vi "FSM_new.vi"() -> ()   [LabVIEW 2016]
panel:
  out "note":string
  out "Waveform Graph 2":dbl[](graph)
  out "Select traing signal":i32
  out "Saved Target":fxp<+/-,32,8>[][](array[numeric])
  out "Number of Signals":i32
  out "Signal Captured":fxp<+/-,32,8>[][](array[numeric])
  in  "Signal Capture":bool
  out "Final Error":fxp<+/-,32,8>
  out "Waveform Graph":dbl[](graph)
  in  "Inference":bool
  in  "Training":bool
  out "Enum":T1(ring)
  out "Weights_oX":fxp<+/-,32,8>[][](array[numeric])
  out "Weights_hX":fxp<+/-,32,8>[][](array[numeric])
  out "Outputs_oX":fxp<+/-,32,8>[](array[numeric])
  out "Outputs_hX":fxp<+/-,32,8>[](array[numeric])
  in  "Target 6":fxp<+/-,32,8>
  in  "Target 5":fxp<+/-,32,8>
  in  "Target 7":fxp<+/-,32,8>
  in  "Target 8":fxp<+/-,32,8>
  in  "Learning rate":fxp<+/-,32,8>
  in  "Offset 2":fxp<+/-,32,8>
  in  "Offset 1":fxp<+/-,32,8>
  out "Random values generated":bool
  out "Training end":bool
  in  "Target 4":fxp<+/-,32,8>
  in  "Target 3":fxp<+/-,32,8>
  in  "Target 2":fxp<+/-,32,8>
  in  "Target 1":fxp<+/-,32,8>
  in  "Stop":bool
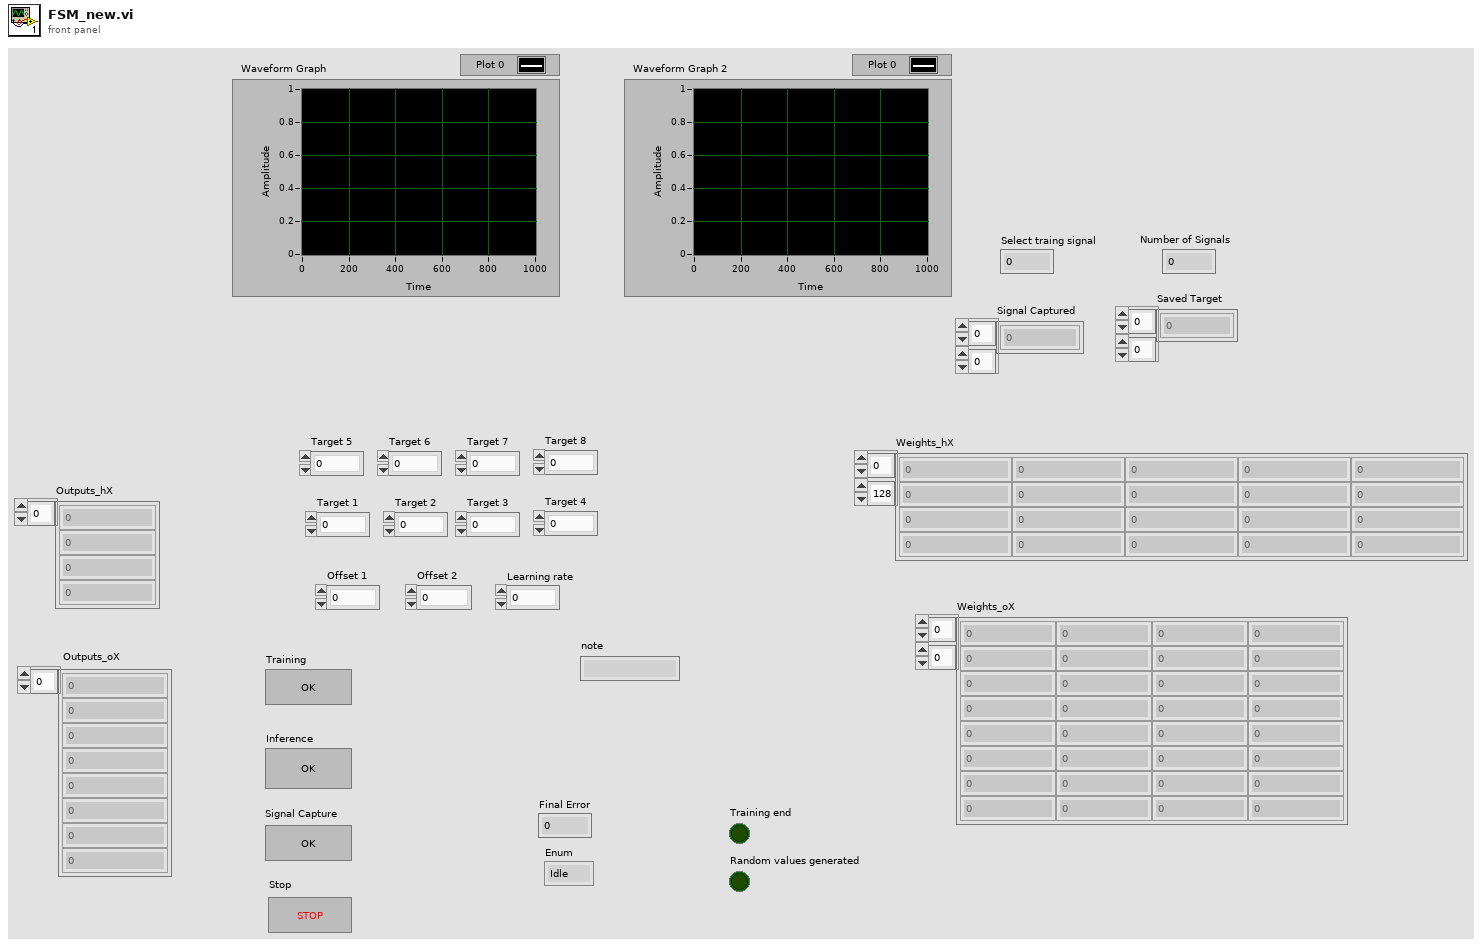
[diagram p1: front panel]
types:
  T1 = enum16{"Idle", "Generate weights", "Training mode", "Inference mode"}
  T2 = enum16{"Idle", "Generate weights", "Training mode", "Inference mode", "Signal Capture"}
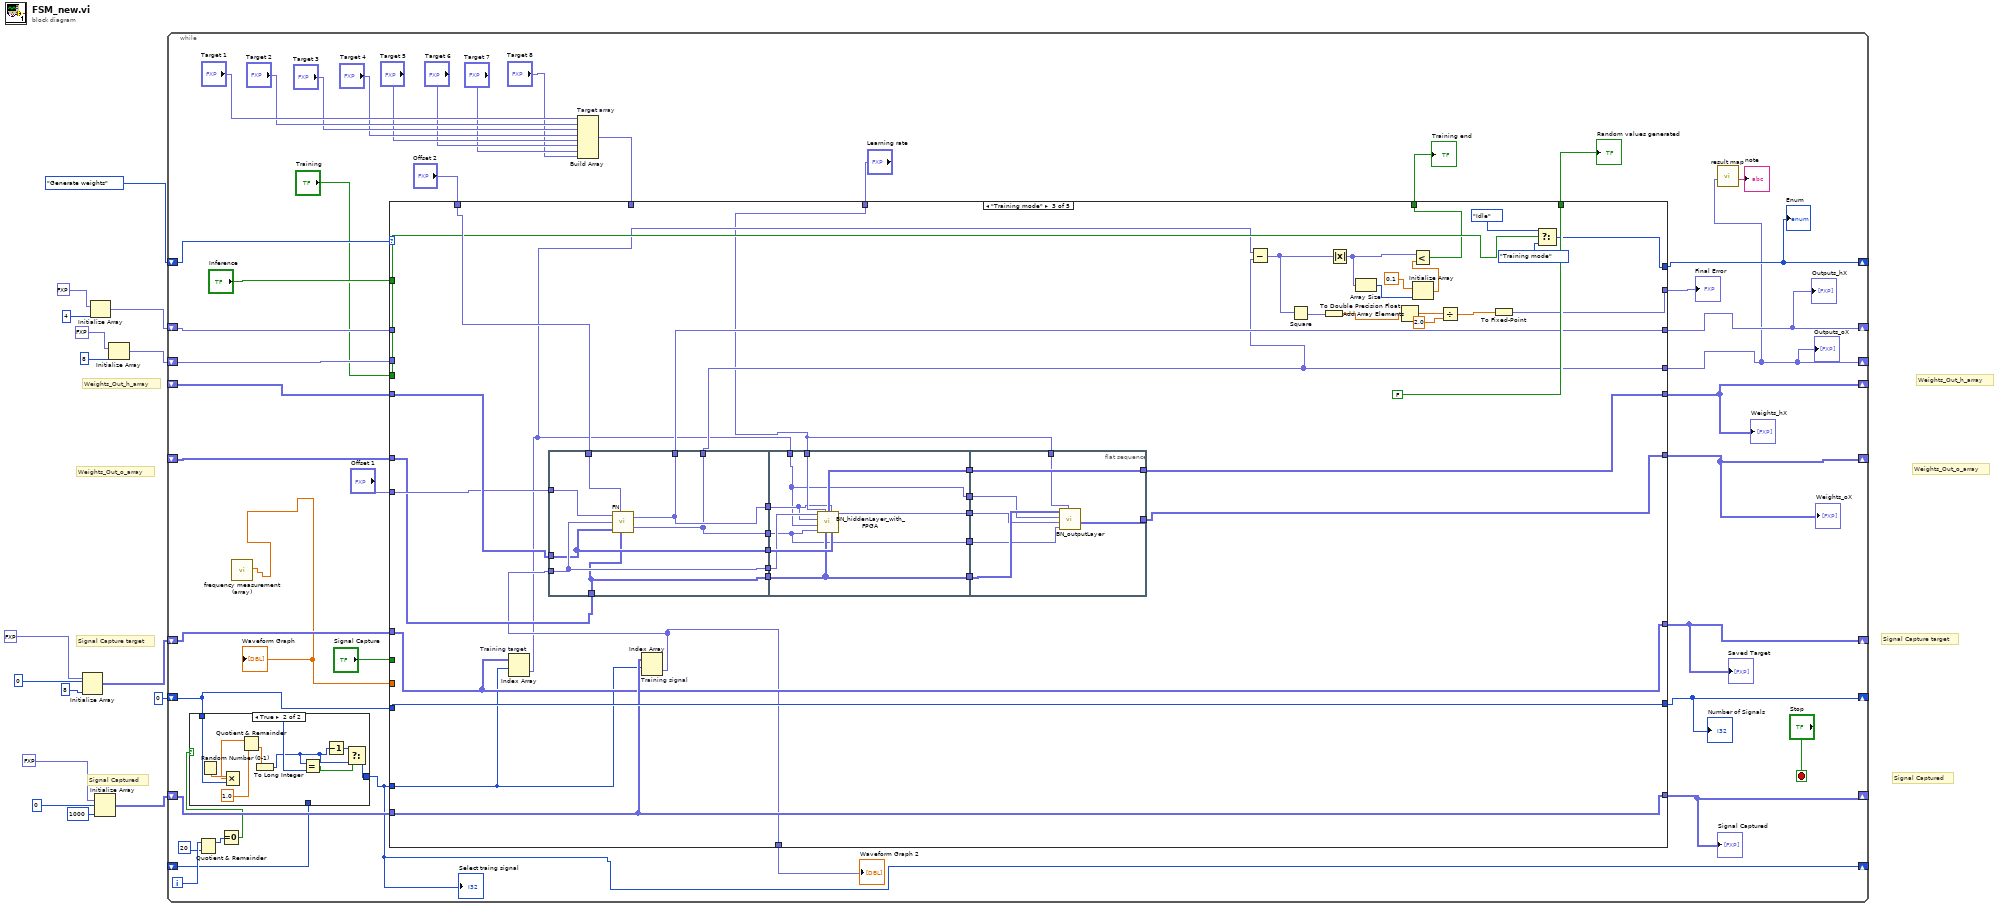
[diagram p0: block diagram]
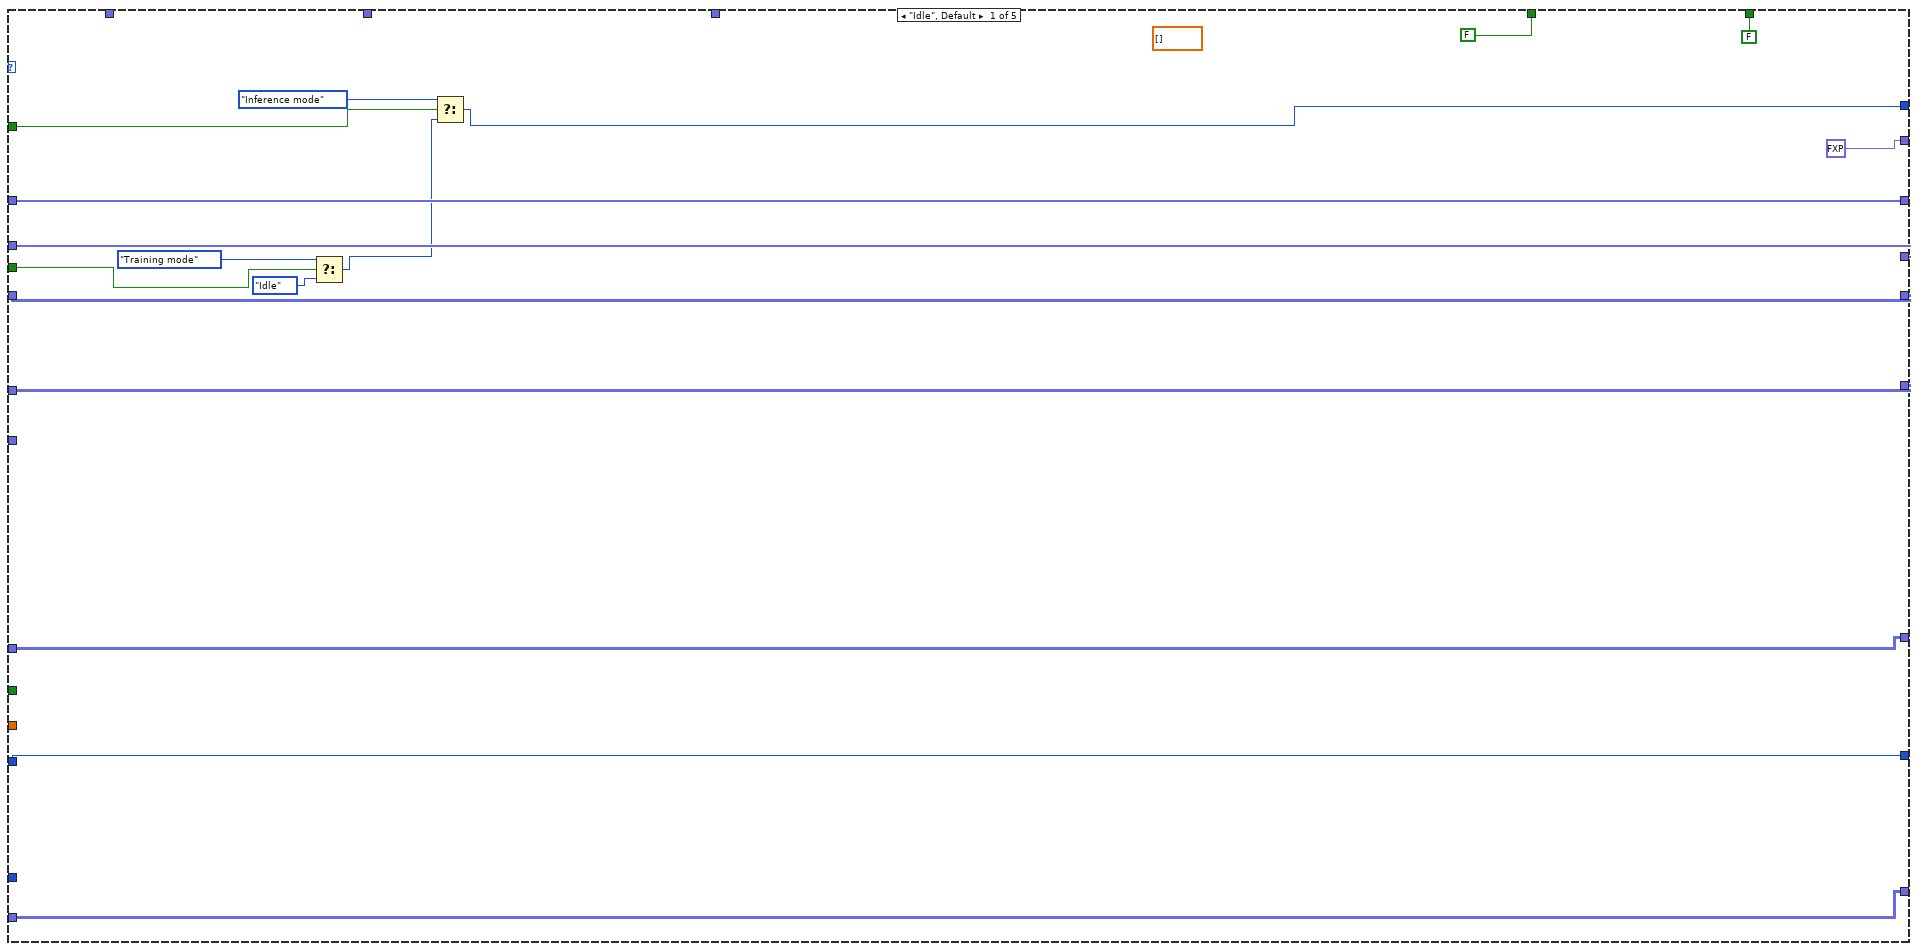
[diagram p3: hidden frame]
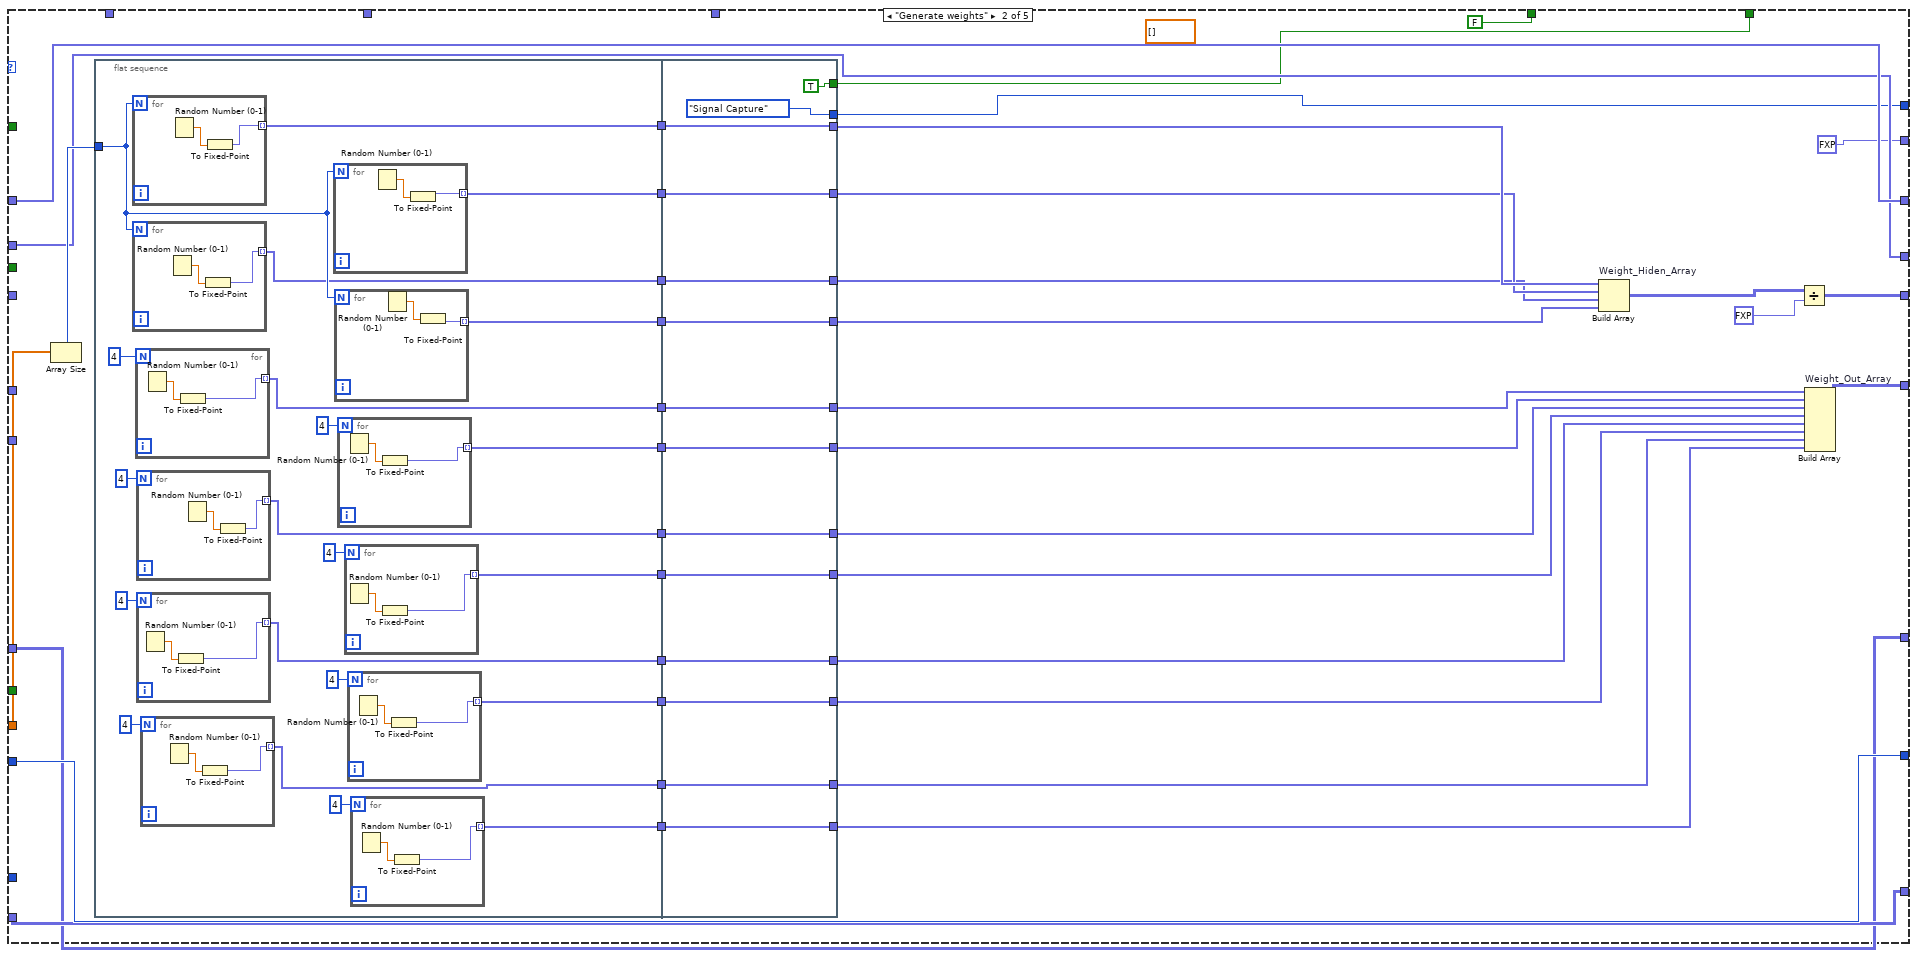
[diagram p4: hidden frame]
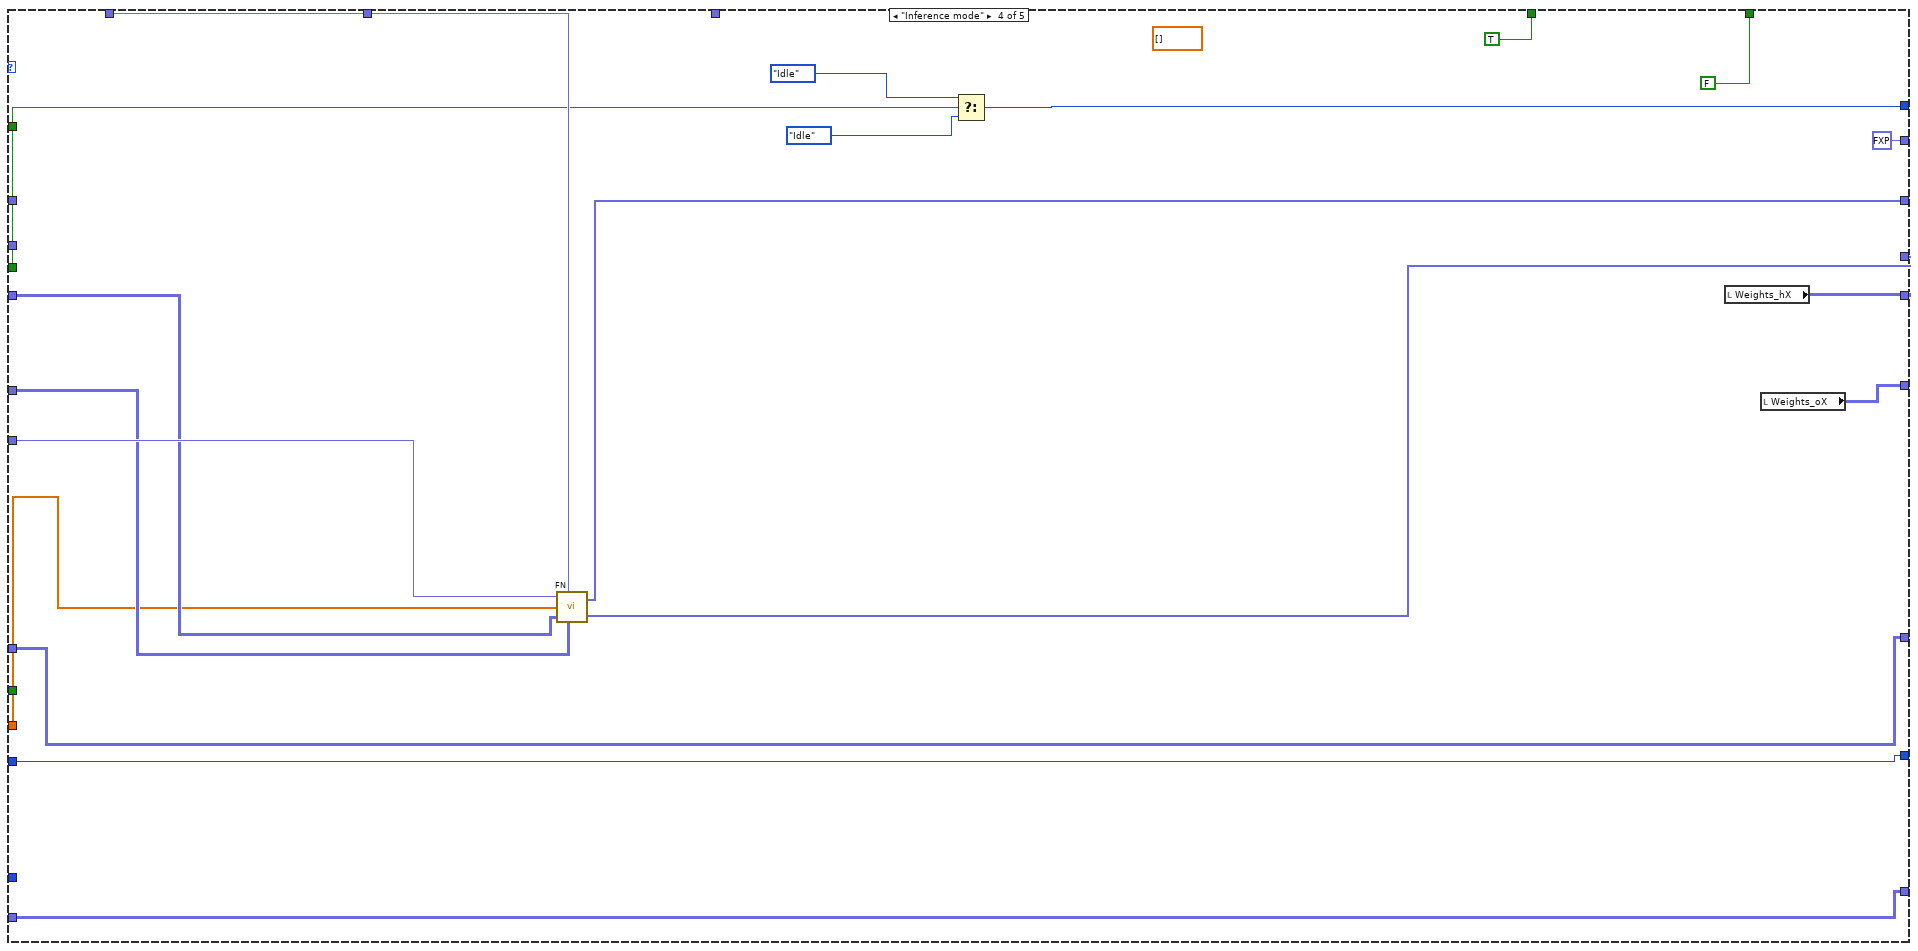
[diagram p5: hidden frame]
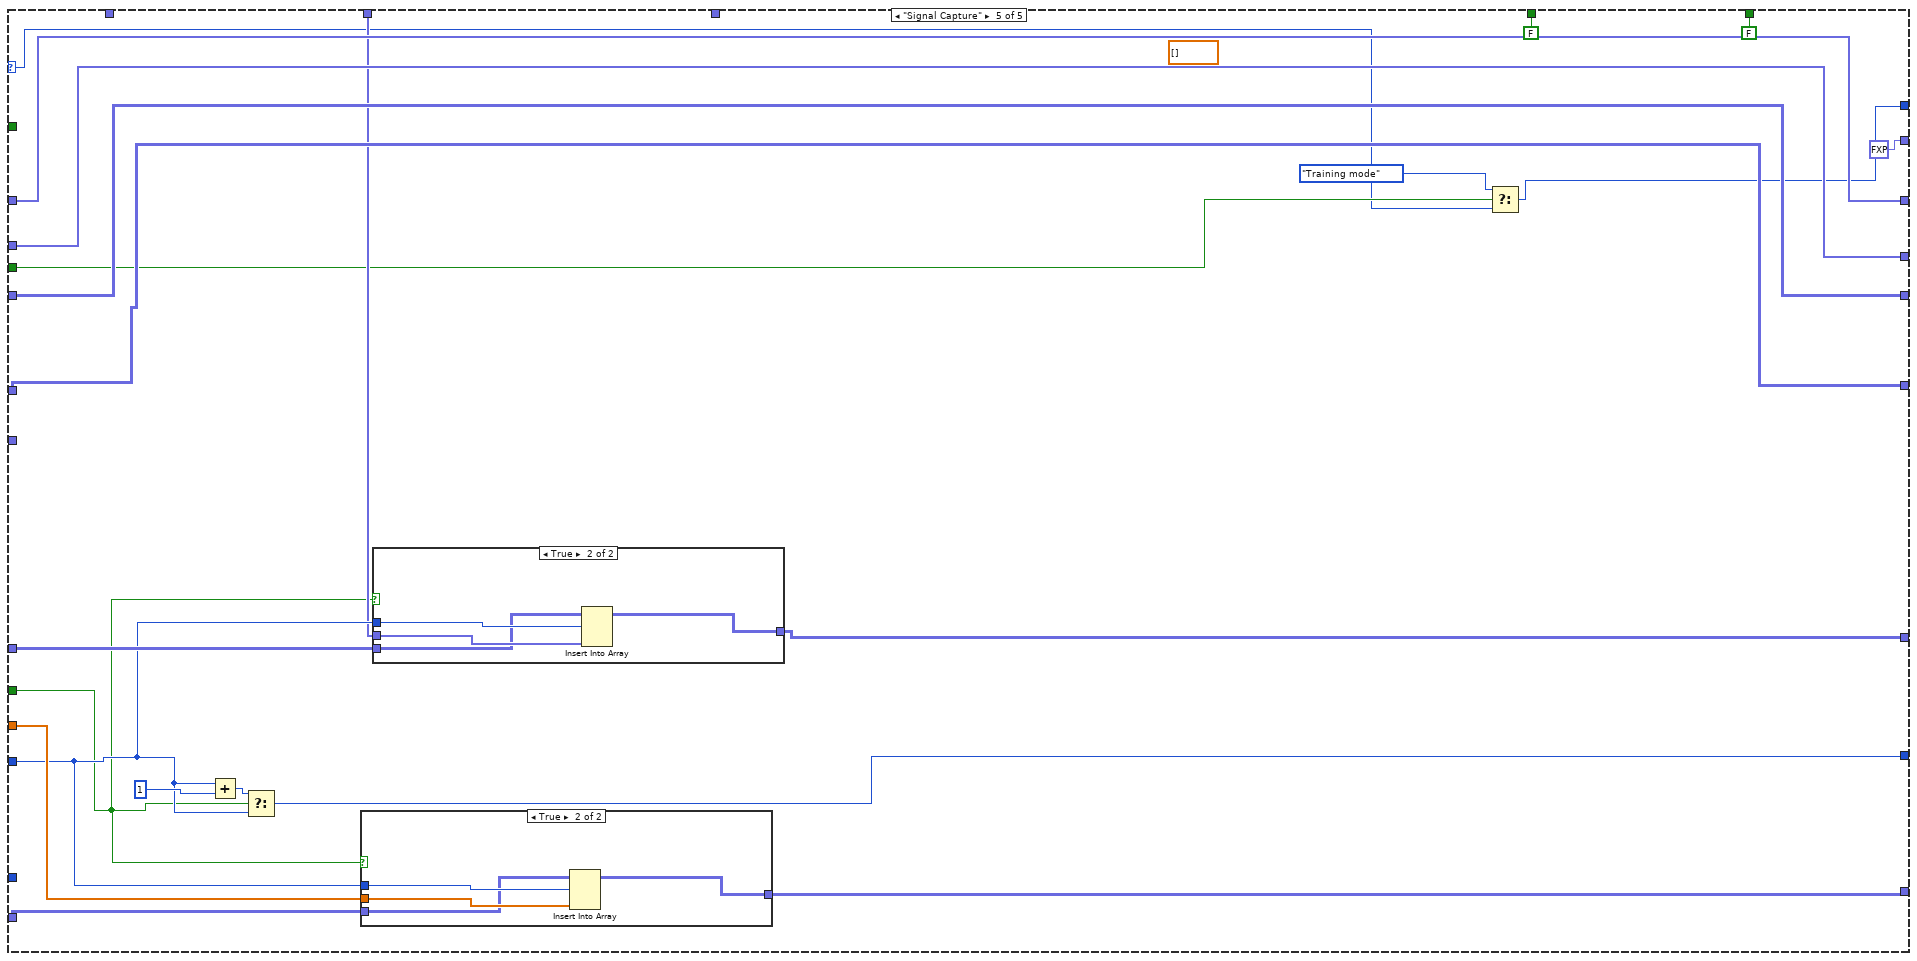
[diagram p6: hidden frame]
diagram:
  # "Signal Captured"
  # "Signal Capture target"
  # "Signal Captured"
  # "Signal Capture target"
  # "Weights_Out_o_array"
  # "Weights_Out_h_array"
  # "Weights_Out_o_array"
  # "Weights_Out_h_array"
  n1 = Initialize Array(fxp<+,32,8> 0.0, 0, 8 ("dimension size")) -> (w1:fxp<+,32,8>[][])
  n2 = Initialize Array(fxp<+,32,8> 0.0, 4) -> (w15:fxp<+,32,8>[])
  n3 = Initialize Array(fxp<+/-,32,8> 0.0, 0, 1000 ("dimension size")) -> (w6:fxp<+/-,32,8>[][])
  n4 = Initialize Array(fxp<+,32,8> 0.0, 8) -> (w10:fxp<+,32,8>[])
  n5 = while {
    shift-right: [w39] -> _
    shift-left: T2."Generate weights" -> [w56]
    shift-right: [w44] -> _
    shift-left: _ -> [w43]
    shift-right: [w45] -> _
    shift-left: _ -> [w42]
    shift-right: [w38] -> _
    shift-left: w15 -> [w41]
    shift-right: [w18] -> _
    shift-left: w10 -> [w40]
    shift-right: [w32] -> _
    shift-left: 0 -> [w25]
    shift-right: [w31] -> _
    shift-left: w6 -> [w30]
    shift-right: [w28] -> _
    shift-left: w1 -> [w29]
    shift-right: [w19] -> _
    shift-left: _ -> [w20]
    i -> [w24]
    stop <- "Stop" stop-if-true
    n6 = Quotient & Remainder(x=w24, y=20) -> (x-y*floor(x/y)=w22:i32)  [unwired: 1 out]
    n7 = Equal To 0?(x=w22) -> (x = 0?=w21:bool)
    n8 = case shown="True" w21 {
      tunnel: w25 -> [_ w66]
      tunnel: [w61 w62] -> w19
      tunnel: w20 -> [w61 _]
      frame False {
      }
      frame True {
        n9 = Random Number (0-1)() -> (number: 0 to 1=w70:dbl)
        n10 = Multiply(x=w70, y=w66) -> (x*y=w69:dbl)
        n11 = Quotient & Remainder(x=w69, y=1.0) -> (floor(x/y)=w67:dbl)  [unwired: 1 out]
        n12 = To Long Integer(number=w67) -> (32bit integer=w63:i32)
        n13 = Equal?(x=w63, y=w66) -> (x = y?=w65:bool)
        n14 = Decrement(x=w63) -> (x-1=w64:i32)
        n15 = Select(t=w64, s=w65, f=w63) -> (s? t:f=w62:i32)
      }
    }
    "Select traing signal" <- w19
    n16 = call "frequency measurement (array).vi"() -> ("real part of fft array"=w26:dbl[])  [unwired: 11 in]
    "Waveform Graph" <- w26
    n17 = Build Array "Target array"("Target 1", "Target 2", "Target 3", "Target 4", "Target 5", "Target 6", "Target 7", "Target 8") -> (w47:fxp<+/-,32,8>[])
    n18 = case shown="\"Training mode\"" w56 {
      selector: w56 -> [_ _ _ _ w271]
      tunnel: [w75 w89 w214 w257 w273] -> w39
      tunnel: [FALSE w97 FALSE FALSE FALSE] -> w46
      tunnel: "Offset 1" -> [_ _ w225 w267 _]
      tunnel: "Offset 2" -> [_ _ w224 w268 _]
      tunnel: "Learning rate" -> [_ _ w190 _ _]
      tunnel: w47 -> [_ _ _ _ w276]
      tunnel: [w83 w100 w223 w266 w290] -> w38
      tunnel: [w82 w99 w217 w265 w289] -> w18
      tunnel: w26 -> [_ w98 _ w254 w281]
      tunnel: [w85 w94 w198 w263 w288] -> w44
      tunnel: [w84 w101 w186 w262 w287] -> w45
      tunnel: w43 -> [w85 _ w226 w261 w288]
      tunnel: w42 -> [w84 _ w205 w260 w287]
      tunnel: w41 -> [w83 w100 _ _ w290]
      tunnel: w40 -> [w82 w99 _ _ w289]
      tunnel: "Training" -> [w80 _ w209 w256 w272]
      tunnel: [FALSE FALSE w208 TRUE FALSE] -> w37
      tunnel: "Inference" -> [w77 _ _ _ _]
      tunnel: [fxp<+,32,8> 0.0 fxp<+,32,8> 0.0 w197 fxp<+,32,8> 0.0 fxp<+,32,8> 0.0] -> w34
      tunnel: "Signal Capture" -> [_ _ _ _ w275]
      tunnel: [w73 w92 w204 w252 w282] -> w32
      tunnel: w25 -> [w73 w92 w204 w252 w277]
      tunnel: [w74 w91 w203 w251 w280] -> w31
      tunnel: w30 -> [w74 w91 w203 w251 w279]
      tunnel: w29 -> [w72 w90 w202 w250 w278]
      tunnel: [w72 w90 w202 w250 w274] -> w28
      tunnel: w19 -> [_ _ w199 _ _]
      tunnel: [_ _ w201 _ _] -> w27
      frame "Idle", Default {
        (unwired) dbl[] [] ("Error_out")
        n19 = Select(t=T1."Training mode", s=w80, f=T1."Idle") -> (s? t:f=w76:T1)
        n20 = Select(t=T1."Inference mode", s=w77, f=w76) -> (s? t:f=w75:T1)
      }
      frame "Generate weights" {
        (unwired) dbl[] [] ("Error_out")
        n21 = Array Size(array=w98) -> (size(s)=w126:i32)
        n22 = flat-sequence {
          tunnel: w126 -> [w147]
          tunnel: [w146] -> w125
          tunnel: [w145] -> w124
          tunnel: [w144] -> w123
          tunnel: [w143] -> w122
          tunnel: [w142] -> w121
          tunnel: [w141] -> w120
          tunnel: [w140] -> w119
          tunnel: [w139] -> w118
          tunnel: [w138] -> w117
          tunnel: [w137] -> w116
          tunnel: [w136] -> w115
          tunnel: [w135] -> w114
          tunnel: [TRUE] -> w97
          tunnel: w125 -> [w184]
          tunnel: [w184] -> w113
          tunnel: w124 -> [w183]
          tunnel: [w183] -> w111
          tunnel: w123 -> [w182]
          tunnel: [w182] -> w102
          tunnel: w122 -> [w181]
          tunnel: [w181] -> w104
          tunnel: w121 -> [w180]
          tunnel: [w180] -> w106
          tunnel: w120 -> [w179]
          tunnel: [w179] -> w108
          tunnel: w119 -> [w178]
          tunnel: [w178] -> w112
          tunnel: w118 -> [w177]
          tunnel: [w177] -> w110
          tunnel: w117 -> [w176]
          tunnel: [w176] -> w103
          tunnel: w116 -> [w175]
          tunnel: [w175] -> w105
          tunnel: [w174] -> w107
          tunnel: w115 -> [w174]
          tunnel: w114 -> [w173]
          tunnel: [w173] -> w109
          tunnel: [T2."Signal Capture"] -> w89
          frame #0 {
            n23 = for {
              N: w147 -> [_]
              tunnel: [w170] -> w146 mode=indexing
              n24 = Random Number (0-1)() -> (number: 0 to 1=w171:dbl)
              n25 = To Fixed-Point(number=w171) -> (fixed-point=w170:fxp<+/-,32,8>)  [unwired: 1 in]
            }
            n26 = for {
              N: w147 -> [_]
              tunnel: [w168] -> w145 mode=indexing
              n27 = Random Number (0-1)() -> (number: 0 to 1=w169:dbl)
              n28 = To Fixed-Point(number=w169) -> (fixed-point=w168:fxp<+/-,32,8>)  [unwired: 1 in]
            }
            n29 = for {
              N: 4 -> [_]
              tunnel: [w166] -> w144 mode=indexing
              n30 = Random Number (0-1)() -> (number: 0 to 1=w167:dbl)
              n31 = To Fixed-Point(number=w167) -> (fixed-point=w166:fxp<+/-,32,8>)  [unwired: 1 in]
            }
            n32 = for {
              N: 4 -> [_]
              tunnel: [w158] -> w143 mode=indexing
              n33 = Random Number (0-1)() -> (number: 0 to 1=w159:dbl)
              n34 = To Fixed-Point(number=w159) -> (fixed-point=w158:fxp<+/-,32,8>)  [unwired: 1 in]
            }
            n35 = for {
              N: 4 -> [_]
              tunnel: [w162] -> w142 mode=indexing
              n36 = Random Number (0-1)() -> (number: 0 to 1=w163:dbl)
              n37 = To Fixed-Point(number=w163) -> (fixed-point=w162:fxp<+/-,32,8>)  [unwired: 1 in]
            }
            n38 = for {
              N: 4 -> [_]
              tunnel: [w164] -> w141 mode=indexing
              n39 = Random Number (0-1)() -> (number: 0 to 1=w165:dbl)
              n40 = To Fixed-Point(number=w165) -> (fixed-point=w164:fxp<+/-,32,8>)  [unwired: 1 in]
            }
            n41 = for {
              N: w147 -> [_]
              tunnel: [w160] -> w140 mode=indexing
              n42 = Random Number (0-1)() -> (number: 0 to 1=w161:dbl)
              n43 = To Fixed-Point(number=w161) -> (fixed-point=w160:fxp<+/-,32,8>)  [unwired: 1 in]
            }
            n44 = for {
              N: w147 -> [_]
              tunnel: [w156] -> w139 mode=indexing
              n45 = Random Number (0-1)() -> (number: 0 to 1=w157:dbl)
              n46 = To Fixed-Point(number=w157) -> (fixed-point=w156:fxp<+/-,32,8>)  [unwired: 1 in]
            }
            n47 = for {
              N: 4 -> [_]
              tunnel: [w154] -> w138 mode=indexing
              n48 = Random Number (0-1)() -> (number: 0 to 1=w155:dbl)
              n49 = To Fixed-Point(number=w155) -> (fixed-point=w154:fxp<+/-,32,8>)  [unwired: 1 in]
            }
            n50 = for {
              N: 4 -> [_]
              tunnel: [w152] -> w137 mode=indexing
              n51 = Random Number (0-1)() -> (number: 0 to 1=w153:dbl)
              n52 = To Fixed-Point(number=w153) -> (fixed-point=w152:fxp<+/-,32,8>)  [unwired: 1 in]
            }
            n53 = for {
              N: 4 -> [_]
              tunnel: [w150] -> w136 mode=indexing
              n54 = Random Number (0-1)() -> (number: 0 to 1=w151:dbl)
              n55 = To Fixed-Point(number=w151) -> (fixed-point=w150:fxp<+/-,32,8>)  [unwired: 1 in]
            }
            n56 = for {
              N: 4 -> [_]
              tunnel: [w148] -> w135 mode=indexing
              n57 = Random Number (0-1)() -> (number: 0 to 1=w149:dbl)
              n58 = To Fixed-Point(number=w149) -> (fixed-point=w148:fxp<+/-,32,8>)  [unwired: 1 in]
            }
          }
          frame #1 {
          }
        }
        n59 = Build Array "Weight_Hiden_Array"(w113, w112, w111, w110) -> (w95:fxp<+/-,32,8>[][])
        n60 = Divide(x=w95, y=fxp<+,32,8> 1.0) -> (x/y=w94:fxp<+/-,64,32>[][])
        n61 = Build Array "Weight_Out_Array"(w102, w103, w104, w105, w106, w107, w108, w109) -> (w101:fxp<+/-,32,8>[][])
      }
      frame "Training mode" {
        n62 = Index Array "Training target"(array=w202, index (row)=w199) -> (element=w200:fxp<+,32,8>[])  [unwired: 1 in]
        n63 = flat-sequence {
          tunnel: w201 -> [w232]
          tunnel: w226 -> [w230]
          tunnel: w205 -> [w229]
          tunnel: w225 -> [w234]
          tunnel: w224 -> [w233]
          tunnel: [w231] -> w223
          tunnel: [w228] -> w217
          tunnel: [w232] -> w222
          tunnel: [w231] -> w221
          tunnel: [w228] -> w220
          tunnel: [w230] -> w219
          tunnel: [w229] -> w218
          tunnel: w190 -> [w240]
          tunnel: w222 -> [w241]
          tunnel: w221 -> [w236]
          tunnel: w200 -> [w235]
          tunnel: w220 -> [w237]
          tunnel: w219 -> [w242]
          tunnel: w218 -> [w238]
          tunnel: [w239] -> w192
          tunnel: [w238] -> w191
          tunnel: [w237] -> w189
          tunnel: [w236] -> w188
          tunnel: [w235] -> w187
          tunnel: [w249] -> w198
          tunnel: w192 -> [w249]
          tunnel: w191 -> [w247]
          tunnel: w190 -> [w248]
          tunnel: w189 -> [w244]
          tunnel: w188 -> [w245]
          tunnel: w187 -> [w246]
          tunnel: [w243] -> w186
          frame #0 {
            n64 = call "FN.vi"("Offset_h"=w234, "Offset_out"=w233, "Inputs"=w232, "Weights_h"=w230, "Weights_out"=w229) -> ("Outputs_hx"=w231:fxp<+/-,32,8>[], "Outputs_out"=w228:fxp<+/-,32,8>[])
          }
          frame #1 {
            n65 = call "BN_hiddenLayer_with_FPGA.vi"("Weights_hX_IN"=w242, "Weights_outX(before being updated)"=w238, "Learning rate"=w240, "Out_outX"=w237, "Target_outX"=w235, "Out_hx"=w236, "Inputs"=w241) -> ("Weights_hX_OUT"=w239:fxp<+/-,32,8>[][])  [unwired: 3 in]
          }
          frame #2 {
            n66 = call "BN_outputLayer.vi"("Learning rate"=w248, "Out_outX"=w244, "Out_hx"=w245, "Target_outX"=w246, "Weights_outX_IN"=w247) -> ("Weights_outX_OUT"=w243:fxp<+/-,32,8>[][])  [unwired: 6 in]
          }
        }
        n67 = Index Array "Training signal"(array=w203, index (row)=w199) -> (element=w201:fxp<+/-,32,8>[])  [unwired: 1 in]
        n68 = Subtract(x=w200, y=w217) -> (x-y=w193:fxp<+/-,34,10>[])
        n69 = Square(x=w193) -> (x^2=w195:fxp<+,32,8>[])
        n70 = To Double Precision Float(number=w195) -> (double precision float=w194:dbl[])
        n71 = Absolute Value(x=w193) -> (abs(x)=w212:fxp<+,33,9>[])
        n72 = Array Size(array=w212) -> (size(s)=w211:i32)
        n73 = Add Array Elements(numeric array=w194) -> (sum=w207:dbl)
        n74 = Initialize Array(0.1 ("y"), w211) -> (w210:dbl[])
        n75 = Less?(x=w212, y=w210) -> (x < y?=w208:bool)
        n76 = Divide(x=w207, y=2.0) -> (x/y=w196:dbl)
        n77 = To Fixed-Point(number=w196) -> (fixed-point=w197:fxp<+/-,32,8>)  [unwired: 1 in]
        n78 = Select(t=T1."Idle", s=w209, f=T1."Training mode") -> (s? t:f=w214:T1)
      }
      frame "Inference mode" {
        (unwired) dbl[] [] ("Error_out")
        n79 = call "FN.vi"("Offset_h"=w267, "Offset_out"=w268, "Inputs"=w254, "Weights_h"=w261, "Weights_out"=w260) -> ("Outputs_hx"=w266:fxp<+/-,32,8>[], "Outputs_out"=w265:fxp<+/-,32,8>[])
        n80 = Select(t=T1."Idle", s=w256, f=T1."Idle") -> (s? t:f=w257:T1)
        n81 = local read "Weights_hX"() -> (w263:fxp<+/-,32,8>[][])
        n82 = local read "Weights_oX"() -> (w262:fxp<+/-,32,8>[][])
      }
      frame "Signal Capture" {
        (unwired) dbl[] [] ("Error_out")
        n83 = Add(x=w277, y=1) -> (x+y=w284:i32)
        n84 = Select(t=w284, s=w275, f=w277) -> (s? t:f=w282:i32)
        n85 = case shown="True" w275 {
          tunnel: w277 -> [_ w300]
          tunnel: w281 -> [_ w299]
          tunnel: [w296 w298] -> w280
          tunnel: w279 -> [w296 w297]
          frame False {
          }
          frame True {
            n86 = Insert Into Array(array=w297, index (row)=w300, new element=w299) -> (w298:fxp<+/-,32,8>[][])  [unwired: 1 in]
          }
        }
        n87 = case shown="True" w275 {
          tunnel: w277 -> [_ w295]
          tunnel: w276 -> [_ w294]
          tunnel: [w291 w293] -> w274
          tunnel: w278 -> [w291 w292]
          frame False {
          }
          frame True {
            n88 = Insert Into Array(array=w292, index (row)=w295, new element=w294) -> (w293:fxp<+,32,8>[][])  [unwired: 1 in]
          }
        }
        n89 = Select(t=T2."Training mode", s=w272, f=w271) -> (s? t:f=w273:T2)
      }
    }
    "Weights_hX" <- w44
    "Weights_oX" <- w45
    "Random values generated" <- w46
    "Enum" <- w39
    "Outputs_hX" <- w38
    "Outputs_oX" <- w18
    "Training end" <- w37
    "Final Error" <- w34
    "Number of Signals" <- w32
    "Signal Captured" <- w31
    "Saved Target" <- w28
    "Waveform Graph 2" <- w27
    n90 = call "result map.vi"("output"=w18) -> ("note"=→"note":string)  [unwired: 10 in]
  }
